vi "ConfigureWfrm.vi"(8 "error in (no error)":errorcluster, 10 "SampleRate":dbl=1000.0, 11 "StandardFunction in":refnum<class "StandardFunction.lvclass">) -> (0 "error out":errorcluster, 3 "StandardFunction out":refnum<class "StandardFunction.lvclass">)   [LabVIEW 2014, in "Functions.lvlib" / "StandardFunction.lvclass"]
uses:
  StandardFunction.lvclass
  StandardFunction.lvclass/StandardFunction.ctl
  FunctionBaseClass/FunctionBase.lvclass/FunctionBase.ctl
  Accessors/Read StandardWfrms.vi
  FunctionBaseClass/Accessors/Write Waveforms.vi
  <vilib>/measure/NI_MABase.lvlib
panel:
  out "Waveform Chart":waveform(dbl)[](graph)=[{"t0"=timestamp(0 s since 1904-01-01), "dt"=0.00020833333333333335, "Y"=[0.0, 0.06540312923014306, 0.13052619222005157, 0.19509032201612825, 0.25881904510252074, 0.32143946530316153, 0.3826834323650897, 0.44228869021900125, 0.49999999999999994, 0.5555702330196022, 0.6087614290087205, 0.6593458151000688, 0.7071067811865475, 0.7518398074789774, 0.793353340291235, 0.8314696123025452, 0.8660254037844385, 0.8968727415326883, 0.9238795325112866, 0.9469301294951056, 0.9659258262890682, 0.9807852804032303, 0.9914448613738104, 0.9978589232386034, 1.0, 0.9978589232386034, 0.9914448613738104, 0.9807852804032303, 0.9659258262890683, 0.9469301294951056, 0.9238795325112868, 0.8968727415326883, 0.8660254037844388, 0.8314696123025452, 0.7933533402912354, 0.7518398074789774, 0.7071067811865478, 0.6593458151000688, 0.6087614290087209, 0.5555702330196023, 0.5000000000000002, 0.4422886902190014, 0.38268343236509, 0.32143946530316175, 0.258819045102521, 0.19509032201612847, 0.13052619222005185, 0.06540312923014331, 2.669170223387751e-16, -0.06540312923014278, -0.13052619222005132, -0.19509032201612794, -0.2588190451025205, -0.32143946530316125, -0.38268343236508956, -0.4422886902190009, -0.4999999999999998, -0.5555702330196018, -0.6087614290087204, -0.6593458151000685, -0.7071067811865474, -0.751839807478977, -0.793353340291235, -0.8314696123025449, -0.8660254037844386, -0.896872741532688, -0.9238795325112867, -0.9469301294951055, -0.9659258262890683, -0.9807852804032303, -0.9914448613738105, -0.9978589232386034, -1.0, -0.9978589232386034, -0.9914448613738105, -0.9807852804032303, -0.9659258262890684, -0.9469301294951056, -0.923879532511287, -0.8968727415326883, -0.8660254037844389, -0.8314696123025452, -0.7933533402912355, -0.7518398074789775, -0.7071067811865479, -0.6593458151000691, -0.6087614290087211, -0.5555702330196025, -0.5000000000000004, -0.44228869021900163, -0.3826834323650902, -0.321439465303162, -0.25881904510252124, -0.19509032201612872, -0.13052619222005207, -0.06540312923014356]}, {"t0"=timestamp(0 s since 1904-01-01), "dt"=0.00020833333333333335, "Y"=[-0.8660254037844387, -0.8968727415326884, -0.9238795325112867, -0.9469301294951057, -0.9659258262890682, -0.9807852804032304, -0.9914448613738103, -0.9978589232386035, -0.9999999999999999, -0.9978589232386035, -0.9914448613738103, -0.9807852804032304, -0.9659258262890681, -0.9469301294951056, -0.9238795325112865, -0.8968727415326883, -0.8660254037844384, -0.8314696123025451, -0.7933533402912349, -0.7518398074789773, -0.7071067811865474, -0.6593458151000687, -0.6087614290087205, -0.5555702330196021, -0.49999999999999994, -0.44228869021900113, -0.3826834323650897, -0.3214394653031614, -0.25881904510252074, -0.1950903220161281, -0.1305261922200516, -0.06540312923014292, -4.632253781944318e-17, 0.06540312923014319, 0.13052619222005152, 0.19509032201612836, 0.25881904510252063, 0.32143946530316164, 0.3826834323650896, 0.4422886902190013, 0.49999999999999983, 0.5555702330196022, 0.6087614290087204, 0.6593458151000688, 0.7071067811865474, 0.7518398074789774, 0.7933533402912349, 0.8314696123025452, 0.8660254037844384, 0.8968727415326883, 0.9238795325112865, 0.9469301294951056, 0.9659258262890681, 0.9807852804032303, 0.9914448613738103, 0.9978589232386034, 0.9999999999999999, 0.9978589232386034, 0.9914448613738103, 0.9807852804032303, 0.9659258262890682, 0.9469301294951056, 0.9238795325112867, 0.8968727415326883, 0.8660254037844387, 0.8314696123025452, 0.7933533402912353, 0.7518398074789774, 0.7071067811865477, 0.6593458151000688, 0.6087614290087209, 0.5555702330196022, 0.5000000000000002, 0.44228869021900125, 0.38268343236509, 0.3214394653031616, 0.258819045102521, 0.1950903220161283, 0.13052619222005188, 0.06540312923014313, 3.0540619946201053e-16, -0.06540312923014296, -0.13052619222005127, -0.19509032201612814, -0.2588190451025204, -0.3214394653031614, -0.3826834323650894, -0.4422886902190011, -0.4999999999999996, -0.555570233019602, -0.6087614290087202, -0.6593458151000686, -0.7071067811865471, -0.7518398074789772, -0.7933533402912348, -0.831469612302545]}, {"t0"=timestamp(0 s since 1904-01-01), "dt"=0.00020833333333333335, "Y"=[0.8660254037844387, 0.8314696123025455, 0.7933533402912353, 0.7518398074789776, 0.7071067811865477, 0.6593458151000691, 0.6087614290087209, 0.5555702330196024, 0.5000000000000002, 0.44228869021900147, 0.38268343236509, 0.3214394653031618, 0.258819045102521, 0.19509032201612853, 0.13052619222005188, 0.06540312923014334, 3.11409968992149e-16, -0.06540312923014278, -0.13052619222005127, -0.19509032201612797, -0.2588190451025204, -0.32143946530316125, -0.3826834323650894, -0.44228869021900097, -0.4999999999999996, -0.555570233019602, -0.6087614290087202, -0.6593458151000686, -0.7071067811865471, -0.7518398074789772, -0.7933533402912348, -0.831469612302545, -0.8660254037844384, -0.8968727415326881, -0.9238795325112865, -0.9469301294951056, -0.9659258262890681, -0.9807852804032304, -0.9914448613738103, -0.9978589232386035, -0.9999999999999999, -0.9978589232386035, -0.9914448613738104, -0.9807852804032304, -0.9659258262890683, -0.9469301294951057, -0.9238795325112868, -0.8968727415326884, -0.8660254037844388, -0.8314696123025453, -0.7933533402912354, -0.7518398074789776, -0.7071067811865478, -0.6593458151000692, -0.608761429008721, -0.5555702330196026, -0.5000000000000004, -0.44228869021900175, -0.3826834323650903, -0.3214394653031621, -0.2588190451025213, -0.1950903220161288, -0.13052619222005216, -0.06540312923014363, -5.937497672345304e-16, 0.06540312923014249, 0.130526192220051, 0.1950903220161277, 0.25881904510252013, 0.32143946530316103, 0.3826834323650891, 0.44228869021900075, 0.49999999999999933, 0.5555702330196017, 0.60876142900872, 0.6593458151000684, 0.7071067811865469, 0.7518398074789769, 0.7933533402912346, 0.8314696123025448, 0.8660254037844382, 0.8968727415326879, 0.9238795325112863, 0.9469301294951054, 0.9659258262890679, 0.9807852804032302, 0.99144486137381, 0.9978589232386034, 0.9999999999999998, 0.9978589232386035, 0.9914448613738103, 0.9807852804032305, 0.9659258262890683, 0.9469301294951058, 0.9238795325112868, 0.8968727415326886]}]
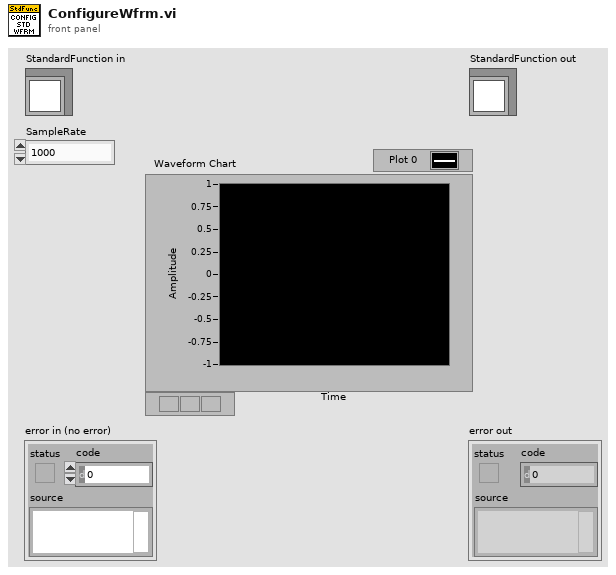
[diagram p1: front panel]
types:
  T1 = enum16{"Sine Wave", "Triangle Wave", "Square Wave", "Sawtooth Wave"}
  T2 = typedef "Functions.lvlib/StandardFunction.lvclass/StdWfrms.ctl" = cluster{"Count":u16, "StandardWfrm":T3[]}
  T3 = typedef "Functions.lvlib/StandardFunction.lvclass/StdWfrm.ctl" = cluster{"Amplitude":dbl, "DcOffset":dbl, "DutyCycle":dbl, "Frequency":dbl, "Phase":dbl, "Waveform":enum16{"Sine", "Square", "Triangle", "Ramp Up", "Ramp Down", "DC"}, "Handle":string}
  T4 = enum16{"Sine", "Square", "Triangle", "Ramp Up", "Ramp Down", "DC"}
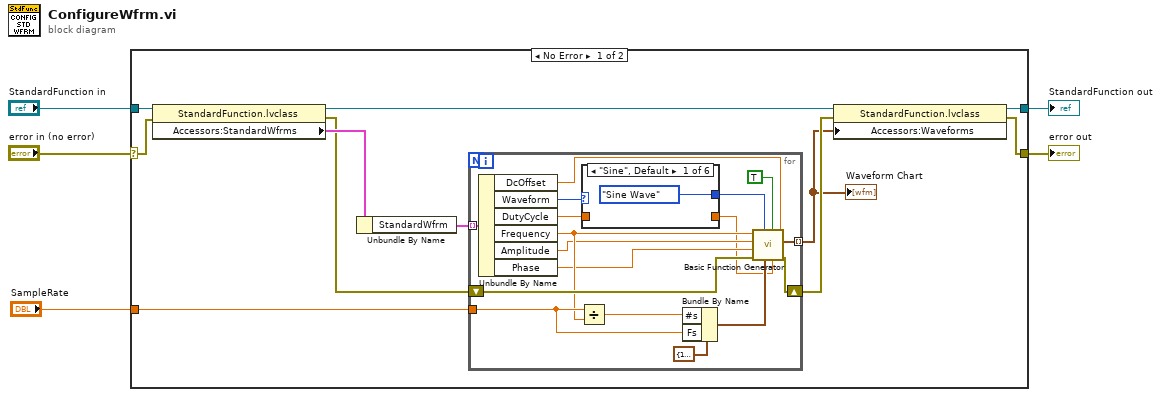
[diagram p0: block diagram]
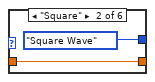
[diagram p2: hidden frame]
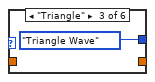
[diagram p3: hidden frame]
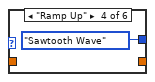
[diagram p4: hidden frame]
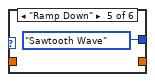
[diagram p5: hidden frame]
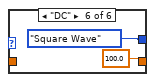
[diagram p6: hidden frame]
diagram:
  n1 = case shown="No Error" "error in (no error)" {
    selector: "error in (no error)" -> [w9 w43]
    tunnel: [w8 w43] -> w4
    tunnel: [w11 w42] -> w2
    tunnel: "StandardFunction in" -> [w16 w42]
    tunnel: "SampleRate" -> [w12 _]
    frame No Error {
      n2 = property class="StandardFunction.lvclass"(reference=w16, error in=w9) -> (reference out=w15:refnum<class "StandardFunction.lvclass">, error out=w13:errorcluster, "Accessors:StandardWfrms"=w14:T2)
      n3 = Unbundle By Name(w14) -> ("StandardWfrm"=w7:T3[])
      n4 = for {
        tunnel: w7 -> [w33] mode=indexing
        tunnel: w12 -> [w25]
        tunnel: [w23] -> w6 mode=indexing
        shift-right: [w22] -> w10
        shift-left: w13 -> [w28]
        n5 = Unbundle By Name(w33) -> ("DcOffset"=w29:dbl, "Waveform"=w32:T4, "DutyCycle"=w18:dbl, "Frequency"=w21:dbl, "Amplitude"=w20:dbl, "Phase"=w19:dbl)
        n6 = Divide(x=w25, y=w21) -> (x/y=w26:dbl)
        n7 = case shown="\"Sine\", Default" w32 {
          tunnel: [T1."Sine Wave" ("signal type") T1."Square Wave" ("signal type") T1."Triangle Wave" ("signal type") T1."Sawtooth Wave" ("signal type") T1."Sawtooth Wave" ("signal type") T1."Square Wave" ("signal type")] -> w31
          tunnel: w18 -> [_ w35 _ _ _ _]
          tunnel: [_ w35 _ _ _ 100.0 ("DutyCycle")] -> w17
          frame "Sine", Default {
          }
          frame "Square" {
          }
          frame "Triangle" {
          }
          frame "Ramp Up" {
          }
          frame "Ramp Down" {
          }
          frame "DC" {
          }
        }
        n8 = Bundle By Name(cluster=cluster{"Fs":dbl, "#s":dbl} {"Fs"=1000.0, "#s"=1000.0} ("sampling info"), "#s"=w26, "Fs"=w25) -> (w24:cluster{"Fs":dbl, "#s":dbl})
        n9 = call <vilib>:"Basic Function Generator.vi"("offset"=w29, "square wave duty cycle (%)"=w17, "reset signal"=TRUE, "sampling info"=w24, "signal type"=w31, "error in (no error)"=w28, "phase"=w19, "amplitude"=w20, "frequency"=w21) -> ("error out"=w22:errorcluster, "signal out"=w23:waveform(dbl))  [unwired: 1 out]
      }
      "Waveform Chart" <- w6
      n10 = property class="StandardFunction.lvclass"(reference=w15, error in=w10, "Accessors:Waveforms"=w6) -> (reference out=w11:refnum<class "StandardFunction.lvclass">, error out=w8:errorcluster)
    }
    frame Error {
    }
  }
  "error out" <- w4
  "StandardFunction out" <- w2
